vi "ZCAN_FilterAck.vi"(0 "error in (no error)":errorcluster caption="错误输入（无错误）", 2 "can_index_handle":u64) -> (14 "error out":errorcluster caption="错误输出", 15 "启动滤波成功？":bool, 16 "can_index_handle(out)":u64)   [LabVIEW 2018, in "zlgcan.lvlib"]
doc: "启动滤波"
uses:
  zlgcan.lvlib
  bin/ControlCANFD.dll
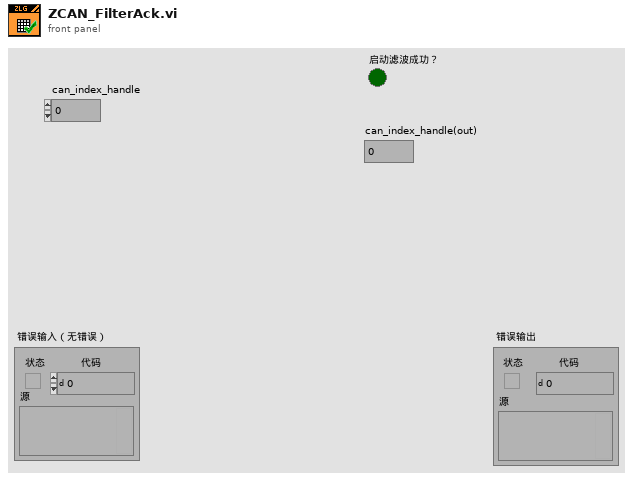
[diagram p1: front panel]
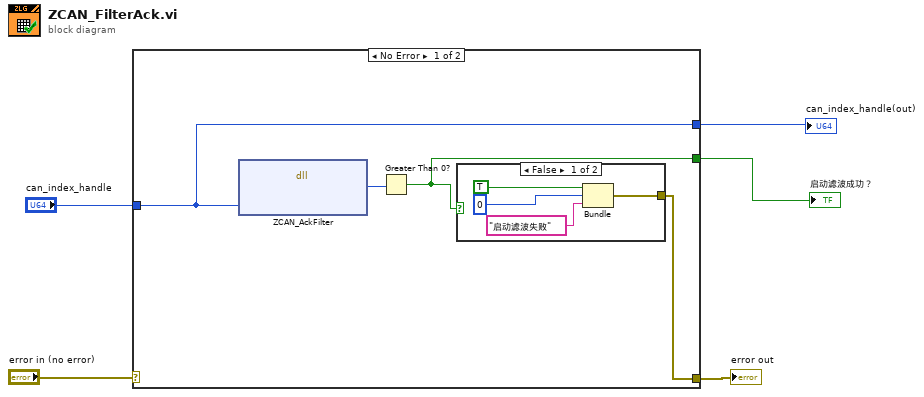
[diagram p0: block diagram]
diagram:
  n1 = case shown="No Error" "error in (no error)" {
    selector: "error in (no error)" -> [_ w14]
    tunnel: [w9 w14] -> w4
    tunnel: "can_index_handle" -> [w8 _]
    tunnel: [w8 _] -> w2
    tunnel: [w6 _] -> w1
    frame No Error {
      n2 = dll-call lib="C:/Users/ttc52/Desktop/DHC FD LV2018/LABIVIEW CANFD Tool_V1.2.4_20220724/bin/ControlCANFD.dll" fn="ZCAN_AckFilter"("channel_handle"=w8) -> ("return"=w7:u32)  [unwired: 4 in, 2 out]
      n3 = Greater Than 0?(x=w7) -> (x > 0?=w6:bool)
      n4 = case shown="False" w6 {
        tunnel: [w10 _] -> w9
        frame False {
          n5 = Bundle("status"=TRUE, "code"=0, "消息"="启动滤波失败") -> (w10:cluster{"status":bool, "code":i32, "消息":string})  [unwired: 1 in]
        }
        frame True {
        }
      }
    }
    frame Error {
    }
  }
  "error out" <- w4
  "can_index_handle(out)" <- w2
  "启动滤波成功？" <- w1
